vi "Release.vi"(8 "error in (no error)":errorcluster, 11 "SequenceFile in":refnum<class "SequenceFile.lvclass">) -> (0 "error out":errorcluster)   [LabVIEW 2020, in "TSnax.lvlib" / "SequenceFile.lvclass"]
uses:
  SequenceFile.lvclass
  SequenceFile.lvclass/SequenceFile.ctl
  PropertyObject/PropertyObject.lvclass/PropertyObject.ctl
  PropertyObject/PropertyObject Ref.vi
  PropertyObjectFile/PropertyObjectFile.lvclass
  C:/dev/illuminated-g/tsnax/TSnax/PropertyObject/PropertyObject.lvclass
  PropertyObject/PropertyObject.lvclass
  Engine/Engine.lvclass
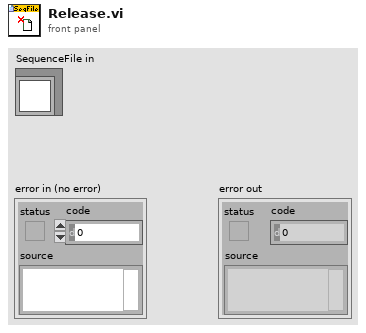
[diagram p1: front panel]
types:
  T1 = typedef "TSnax.lvlib/SequenceFile.lvclass/Ref Data.ctl" = cluster{"Process Model":refnum<class "PropertyObjectFile.lvclass">, "File Globals":refnum<class "PropertyObject.lvclass">}
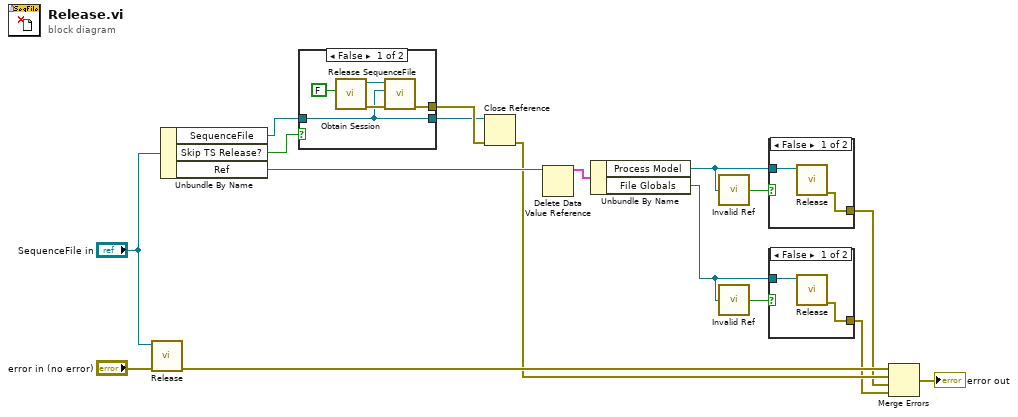
[diagram p0: block diagram]
diagram:
  n1 = call-parent "Release.vi"("error in (no error)"="error in (no error)", "PropertyObject in"="SequenceFile in") -> ("error out"=w9:errorcluster)  [unwired: 9 in]
  n2 = Unbundle By Name("SequenceFile in") -> ("SequenceFile"=w12:refnum<k7>, "Skip TS Release?"=w13:bool, "Ref"=w14:refnum<data-value>)
  n3 = case shown="False" w13 {
    tunnel: w12 -> [w18 w23]
    tunnel: [w19 _] -> w17
    tunnel: [w18 w23] -> w11
    frame False {
      n4 = call "Obtain Session.vi"("Create if needed? (T)"=FALSE) -> ("error out"=w20:errorcluster, "Engine out"=w21:refnum<class "Engine.lvclass">)  [unwired: 9 in]
      n5 = call "Release SequenceFile.vi"("error in (no error)"=w20, "SequenceFile"=w18, "Engine in"=w21) -> ("error out"=w19:errorcluster)  [unwired: 7 in, 1 out]
    }
    frame True {
    }
  }
  n6 = Close Reference(reference=w11, error in (no error)=w17) -> (error out=w3:errorcluster)
  n7 = Delete Data Value Reference(data value reference=w14) -> (data value=w8:T1)  [unwired: 1 in, 1 out]
  n8 = Unbundle By Name(w8) -> ("Process Model"=w6:refnum<class "PropertyObjectFile.lvclass">, "File Globals"=w4:refnum<class "PropertyObject.lvclass">)
  n9 = call "Invalid Ref.vi"("PropertyObject"=w6) -> ("Not a Valid Ref?"=w7:bool)
  n10 = call "Invalid Ref.vi"("PropertyObject"=w4) -> ("Not a Valid Ref?"=w5:bool)
  n11 = case shown="False" w7 {
    tunnel: w6 -> [w25 _]
    tunnel: [w24 _] -> w1
    frame False {
      n12 = call-dynamic "Release.vi"("PropertyObject in"=w25) -> ("error out"=w24:errorcluster)  [unwired: 10 in]
    }
    frame True {
    }
  }
  n13 = case shown="False" w5 {
    tunnel: w4 -> [w27 _]
    tunnel: [w26 _] -> w2
    frame False {
      n14 = call-dynamic "Release.vi"("PropertyObject in"=w27) -> ("error out"=w26:errorcluster)  [unwired: 10 in]
    }
    frame True {
    }
  }
  n15 = Merge Errors(w9, w3, w1, w2) -> (→"error out":errorcluster)
